vi "Read Dual Fan Actor.vi"(11 "蒸发冷却器":refnum<class "Evaporative Cooler.lvclass">) -> (2 "双风扇":refnum<class "Dual Fan.lvclass">)   [LabVIEW 2013, in "Evaporative Cooler.lvlib" / "Evaporative Cooler.lvclass"]
doc: "读取“双风扇”操作者，该操作者应由蒸发冷却器负责启动。子类中必须对该方法进行重写以返回符合应用需要的双风扇。例如，仿真的蒸发冷却器需要返回仿真的双风扇。"
uses:
  Evaporative Cooler.lvclass
  Dual Fan/Dual Fan/Dual Fan.lvclass
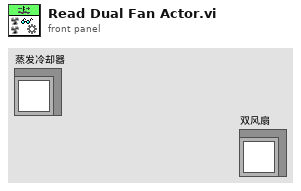
[diagram p1: front panel]
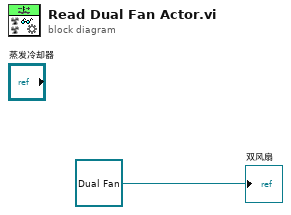
[diagram p0: block diagram]
diagram:
  "双风扇" <- refnum<class "Dual Fan.lvclass"> refnum ("Dual Fan.lvclass")
